vi "LQR.vi"() -> ()   [LabVIEW 2019]
uses:
  <vilib>/Platform/TimedLoop/XDataNode/timing_clust.ctl
  <vilib>/Platform/TimedLoop/XDataNode/nitl_modes.ctl
  <vilib>/Platform/TimedLoop/XDataNode/wakeup.ctl
  <vilib>/Simulation/Shared/_Datatypes/SIM SISO Transfer Function.ctl
  <vilib>/myRIO/Instrument Drivers/Onboard IO/AI/typedefs/AI Reference.ctl
  <vilib>/myRIO/Common/Instrument Driver Framework/Utilities/typedefs/myRIO Generic Hardware Reference.ctl
  <vilib>/myRIO/Common/Instrument Driver Framework/Utilities/typedefs/Hardware Version Enum.ctl
  <vilib>/myRIO/Common/Instrument Driver Framework/Utilities/typedefs/myRIO v1.0 Reference.ctl
  <vilib>/myRIO/Common/Instrument Driver Framework/Utilities/typedefs/Generic FPGA Reference.ctl
  <vilib>/myRIO/Common/Instrument Driver Framework/myRIO v1.0/AI/typedefs/AI Channels List.ctl
  <vilib>/myRIO/Common/Instrument Driver Framework/myRIO v1.0/AI/typedefs/AI Channels Enum.ctl
  <vilib>/myRIO/Common/Instrument Driver Framework/Utilities/typedefs/Analog Scaling Constants List.ctl
  <vilib>/myRIO/Common/Instrument Driver Framework/Utilities/typedefs/Analog Scaling Constants.ctl
  <vilib>/userDefined/High Color/nirio_resource_hc.ctl
  <vilib>/myRIO/Instrument Drivers/Onboard IO/AO/typedefs/AO Reference.ctl
  <vilib>/myRIO/Common/Instrument Driver Framework/myRIO v1.0/AO/typedefs/AO Channels List.ctl
  <vilib>/myRIO/Common/Instrument Driver Framework/myRIO v1.0/AO/typedefs/AO Channels Enum.ctl
  <vilib>/myRIO/Common/Instrument Driver Framework/Utilities/vis/Is FPGA Ref Available.vi
  <vilib>/myRIO/Common/Instrument Driver Framework/myRIO v1.0/AI/vis/myRIO v1.1 Open AI.vi
  <vilib>/myRIO/Instrument Drivers/Onboard IO/AI/vis/Read.vi
  <vilib>/Simulation/DiscreteLinear/Implementation/NILVSim Discrete Transfer Function Direct.llb/SIM Discrete Transfer Function Diagram (SISO).vi
  <vilib>/myRIO/Common/Instrument Driver Framework/myRIO v1.0/AO/vis/myRIO v1.1 Open AO.vi
  <vilib>/myRIO/Instrument Drivers/Onboard IO/AO/vis/Write.vi
  <vilib>/myRIO/Common/Instrument Driver Framework/Utilities/vis/Validate Channels.vi
  <vilib>/myRIO/Common/Instrument Driver Framework/myRIO v1.0/AI/vis/myRIO v1.0 Reserve AI.vi
  <vilib>/Simulation/ContinuousLinear/Implementation/Shared/SIM Transfer Function Support.llb/SIM TransferFunction Normalize to Buffer.vi
  <vilib>/Simulation/DiscreteLinear/Implementation/Shared/SIM Init Discrete States.vi
  <vilib>/Simulation/DiscreteLinear/Implementation/NILVSim Discrete Transfer Function Direct.llb/SIM Transfer Function Direct core (SISO).vi
  <vilib>/myRIO/Common/Instrument Driver Framework/myRIO v1.0/AO/vis/myRIO v1.0 Reserve AO.vi
  <vilib>/myRIO/Common/Instrument Driver Framework/myRIO v1.0/AI/vis/myRIO v1.0 Build MUX Configuration AI.vi
  <vilib>/myRIO/Common/Instrument Driver Framework/myRIO v1.0/Resource Manager/vis/myRIO v1.0 Reserve Channel List.vi
  <vilib>/Simulation/ContinuousLinear/Implementation/Shared/SIM Transfer Function Support.llb/SIM TransferFunction Normalize.vi
  <vilib>/myRIO/Common/Instrument Driver Framework/myRIO v1.0/AO/vis/myRIO v1.0 Build MUX Configuration AO.vi
  <vilib>/myRIO/Common/Instrument Driver Framework/myRIO v1.0/Resource Manager/vis/myRIO v1.0 Reserve Channel.vi
  <vilib>/myRIO/Common/Instrument Driver Framework/myRIO v1.0/Resource Manager/vis/myRIO v1.0 Unreserve Channel.vi
  <vilib>/Simulation/Implementation/Shared/SIM Polynomials.llb/SIM Remove Zero Coefficients (DBL).vi
  <vilib>/myRIO/Common/Instrument Driver Framework/myRIO v1.0/Resource Manager/vis/myRIO v1.0 Build Mutex Name.vi
  <vilib>/Simulation/Implementation/Shared/SIM Polynomials.llb/SIM Divide Polynomials (DBL).vi
  <vilib>/Simulation/Implementation/Shared/SIM BuildSimErr.vi
  <vilib>/Utility/VariantDataType/GetNumericInfo.vi
  <vilib>/Utility/error.llb/Error Cluster From Error Code.vi
  <vilib>/myRIO/Common/Instrument Driver Framework/myRIO v1.0/myRIO v1.1 Open.vi
  <vilib>/myRIO/Common/Instrument Driver Framework/myRIO v1.0/AI/vis/myRIO v1.0 Get Scaling Constants AI.vi
  <vilib>/myRIO/Common/Instrument Driver Framework/Utilities/vis/IO Manager.vi
  <vilib>/myRIO/Common/Instrument Driver Framework/Utilities/vis/Configuration Manager.vi
  <vilib>/myRIO/Common/Instrument Driver Framework/myRIO v1.0/myRIO v1.0 Close.vi
  <vilib>/myRIO/Common/Instrument Driver Framework/myRIO v1.0/AI/vis/myRIO v1.0 Read AI.vi
  <vilib>/myRIO/Common/Instrument Driver Framework/myRIO v1.0/AO/vis/myRIO v1.0 Get Scaling Constants AO.vi
  <vilib>/myRIO/Common/Instrument Driver Framework/myRIO v1.0/AO/vis/myRIO v1.0 Write AO.vi
  <vilib>/platform/TimedLoop/XDataNode/XDataNode.xnode
  <vilib>/Simulation/Implementation/XNodeFramework/SimXNode/SimX.xnode
  <vilib>/myRIO/Express VI/Onboard IO/AI/AI Express VI.xnode
  <vilib>/myRIO/Instrument Drivers/Onboard IO/AI/vis/myRIO AI Open.xnode
  <vilib>/myRIO/Express VI/Onboard IO/AO/AO Express VI.xnode
  <vilib>/myRIO/Instrument Drivers/Onboard IO/AO/vis/myRIO AO Open.xnode
  <vilib>/Platform/TimedLoop/XDataNode/XDNodeRunTimeDep.lvlib
  <vilib>/myRIO/Instrument Drivers/Onboard IO/AI/AI.lvlib
  <vilib>/myRIO/Instrument Drivers/Onboard IO/AO/AO.lvlib
  <vilib>/ptbypt/NI_PtbyPt.lvlib
panel:
  in  "amplitude":dbl=1.0 format="%0.2f"
  out "Impulse Pattern":dbl(graph)
  in  "D":dbl=7.3
  in  "P":dbl=5291.0
  in  "stopNoise":bool=TRUE
  in  "gain_noise":dbl=0.2
  out "uniform white noise":dbl(graph)=-0.031193239239623867
  in  "AmpWhitehNoise":dbl=1.0 format="%0.2f"
  out "Iteration Duration":i64(graph)=347
  in  "Max FRF current 0-1000mA":dbl=4.0
  in  "Stop FRF":bool=TRUE
  in  "esc":bool
  out "scope":cluster{dbl, dbl, dbl, dbl, dbl}(graph)={-8.303163599999976, 0.03990822535355048, -0.0, -8.32082689025263, 946.4168275057085}
  out "Current Output EM":dbl(graph)=0.03990822535355048
  in  "Stop EM + FRF":bool=TRUE
  out "left[V]":dbl=-0.0
  out "right[V]":dbl=-0.0
  out "um":dbl=376.9531636
  # "mA"
types:
  T1 = typedef "XDNodeRunTimeDep.lvlib/timing_clust.ctl" = cluster{"Expected End [f-1]":u64, "Actual End [f-1]":u64, "Finished Late? [f-1]":bool, "Expected End [i-1]":u64, "Actual End [i-1]":u64, "Finished Late? [i-1]":bool, "Expected Start [i]":u64, "Actual Start [i]":u64, "Expected Start [f]":u64, "Actual Start [f]":u64, "Source Name":string, "Structure Name":string, "Period":i64, "Deadline":i64, "Offset":i64, "Start":i64, "Priority":i32, "Timeout":i32, "Mode":T2, "Wakeup Reason":T3, "Error":errorcluster, "Source Type":string, "Secondary Source Type":string, "Global End Time":u64, "Global Start Time":u64, "Frame Duration":u64, "Iteration Duration":u64, "Assigned CPU":i32, "I/O Scan Engine Mode":u32}
  T2 = typedef "XDNodeRunTimeDep.lvlib/nitl_modes.ctl" = enum32{"No Change", "Process missed periods, maintain original phase", "Discard missed periods, maintain original phase", "Process missed periods, ignore original phase", "Discard missed periods, ignore original phase"}
  T3 = typedef "XDNodeRunTimeDep.lvlib/wakeup.ctl" = enum32{"Normal", "Aborted", "Asynchronous wakeup", "Timing source error", "Timed loop error", "Timeout"}
  T4 = typedef "SIM SISO Transfer Function.ctl" = cluster{"Numerator":dbl[], "Denominator":dbl[]}
  T5 = typedef "AI.lvlib/AI Reference.ctl" = cluster{"myRIO Reference":T6, "AI Channels List":T10, "AI Scaling Constants List":T12}
  T6 = typedef "myRIO Generic Hardware Reference.ctl" = cluster{"myRIO Model":T7, "myRIO Hardware Reference":T8}
  T7 = typedef "Hardware Version Enum.ctl" = enum16{"Unknown", "myRIO-1900", "myRIO-1950", "roboRIO", "NI ELVIS RIO CM", "ELVIS III"}
  T8 = typedef "myRIO v1.0 Reference.ctl" = cluster{"Generic FPGA Reference":T9, "Allow multiple opens":bool}
  T9 = typedef "Generic FPGA Reference.ctl" = refnum<k20>
  T10 = typedef "AI Channels List.ctl" = T11[]
  T11 = typedef "AI Channels Enum.ctl" = enum16{"Not Connected", "AudioIn/Left", "AudioIn/Right", "C/AI0", "C/AI1", "A/AI0", "A/AI1", "A/AI2", "A/AI3", "A/AI4", "A/AI5", "A/AI6", "A/AI7", "B/AI0", "B/AI1", "B/AI2", "B/AI3", "B/AI4", "B/AI5", "B/AI6", "B/AI7", "AI/AI0", "AI/AI1", "AI/AI2", "AI/AI3", "A/AI0 (DIFF)", "A/AI1 (DIFF)", "A/AI2 (DIFF)", "A/AI3 (DIFF)", "B/AI0 (DIFF)", "B/AI1 (DIFF)", "B/AI2 (DIFF)", "B/AI3 (DIFF)"}
  T12 = typedef "Analog Scaling Constants List.ctl" = T13[]
  T13 = typedef "Analog Scaling Constants.ctl" = cluster{"LSB Weight (Volts)":dbl, "Offset (Volts)":dbl, "Signed?":bool}
  T14 = typedef "nirio_resource_hc.ctl" = tag
  T15 = typedef "AO.lvlib/AO Reference.ctl" = cluster{"myRIO Reference":T6, "AO Channel List":T16, "AO Scaling Constant List":T12}
  T16 = typedef "AO Channels List.ctl" = T17[]
  T17 = typedef "AO Channels Enum.ctl" = enum16{"Not Connected", "AudioOut/Left", "AudioOut/Right", "C/AO0", "C/AO1", "A/AO0", "A/AO1", "B/AO0", "B/AO1"}
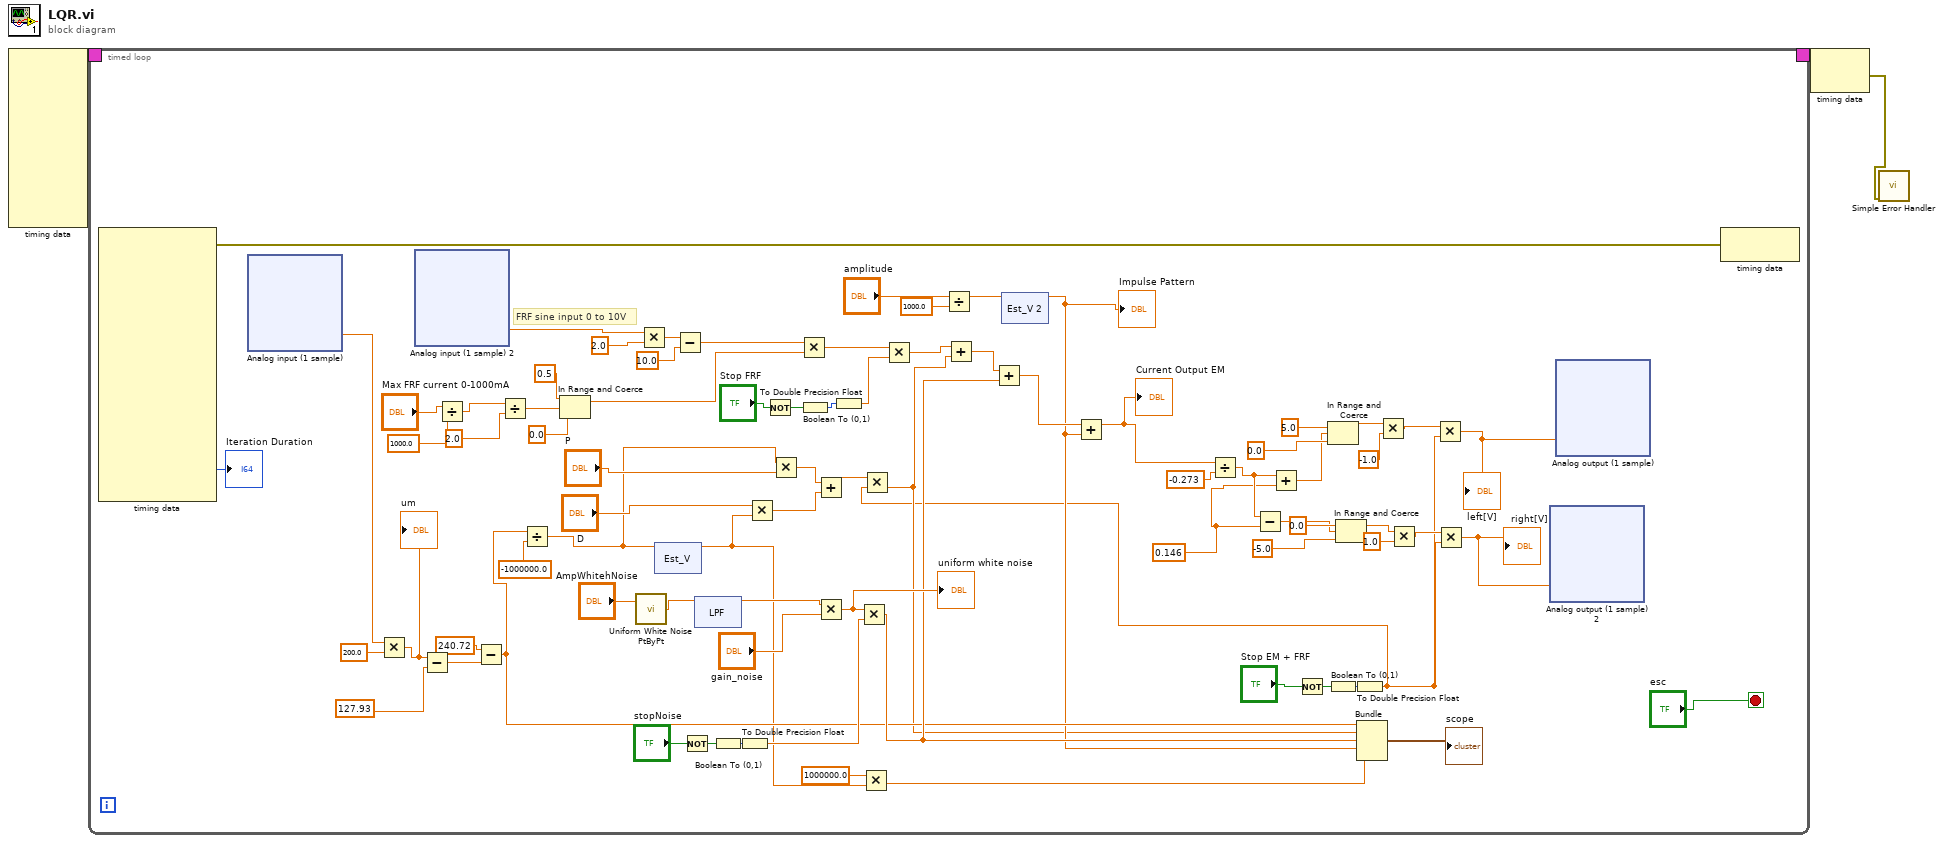
[diagram p0: block diagram]
diagram:
  n1 = node-c288() -> (w3:T1)  [unwired: 10 in]
  n2 = timed-loop {
    timing: w3 -> [_]
    timing-out: [_] -> w2
    stop <- "esc" stop-if-true
    w41 = 0.146 ("y")
    # "FRF sine input 0 to 10V"
    n3 = node-c288() -> (w82:errorcluster, →"Iteration Duration":i64)  [unwired: 1 in, 15 out]
    n4 = xnode "Analog input (1 sample)"() -> ("C/AI1 (AI1)"=w38:dbl)  [unwired: 1 in, 1 out]
    n5 = Multiply(x=w38, y=200.0) -> (x*y=w80:dbl)
    "um" <- w80
    n6 = xnode "Analog input (1 sample) 2"() -> ("C/AI0 (AI0)"=w59:dbl)  [unwired: 1 in, 1 out]
    n7 = Subtract(x=w80, y=127.93) -> (x-y=w79:dbl)
    n8 = Divide(x="Max FRF current 0-1000mA", y=1000.0) -> (x/y=w48:dbl)
    n9 = Subtract(x=240.72, y=w79) -> (x-y=w21:dbl)
    n10 = Divide(x=w48, y=2.0) -> (x/y=w52:dbl)
    n11 = Divide(x=w21, y=-1000000.0) -> (x/y=w11:dbl)
    n12 = In Range and Coerce(upper limit=0.5, x=w52, lower limit=0.0) -> (coerced(x)=w49:dbl)  [unwired: 1 out]
    n13 = call <vilib>:"Uniform White Noise PtByPt.vi"("amplitude"="AmpWhitehNoise") -> ("uniform white noise"=w31:dbl)  [unwired: 2 in]
    n14 = Multiply(x=w59, y=2.0) -> (x*y=w57:dbl)
    n15 = xnode "Est_V"("input u(k)"=w11) -> ("output y(k)"=w12:dbl)  [unwired: 2 in, 1 out]
    n16 = Subtract(x=w57, y=10.0) -> (x-y=w54:dbl)
    n17 = Not(x="stopNoise") -> (.not. x?=w29:bool)
    n18 = xnode "LPF"("input u(k)"=w31) -> ("output y(k)"=w28:dbl)  [unwired: 2 in, 1 out]
    n19 = Boolean To (0,1)(Boolean=w29) -> (0, 1=w30:i16)
    n20 = To Double Precision Float(number=w30) -> (double precision float=w25:dbl)
    n21 = Multiply(x="D", y=w12) -> (x*y=w19:dbl)
    n22 = Not(x="Stop FRF") -> (.not. x?=w62:bool)
    n23 = Multiply(x=w11, y="P") -> (x*y=w20:dbl)
    n24 = Multiply(x=w54, y=w49) -> (x*y=w55:dbl)
    n25 = Boolean To (0,1)(Boolean=w62) -> (0, 1=w61:i16)
    n26 = Add(x=w20, y=w19) -> (x+y=w5:dbl)
    n27 = Multiply(x=w28, y="gain_noise") -> (x*y=w24:dbl)
    "uniform white noise" <- w24
    n28 = To Double Precision Float(number=w61) -> (double precision float=w60:dbl)
    n29 = Multiply(x=w24, y=w25) -> (x*y=w23:dbl)
    n30 = Multiply(x=1000000.0, y=w12) -> (x*y=w8:dbl)
    n31 = Multiply(x=w55, y=w60) -> (x*y=w64:dbl)
    n32 = Divide(x="amplitude", y=1000.0) -> (x/y=w14:dbl)
    n33 = xnode "Est_V 2"("input u(k)"=w14) -> ("output y(k)"=w9:dbl)  [unwired: 2 in, 1 out]
    "Impulse Pattern" <- w9
    n34 = Not(x="Stop EM + FRF") -> (.not. x?=w67:bool)
    n35 = Boolean To (0,1)(Boolean=w67) -> (0, 1=w69:i16)
    n36 = To Double Precision Float(number=w69) -> (double precision float=w4:dbl)
    n37 = Multiply(x=w5, y=w4) -> (x*y=w6:dbl)
    n38 = Add(x=w64, y=w6) -> (x+y=w22:dbl)
    n39 = Add(x=w22, y=w23) -> (x+y=w16:dbl)
    n40 = Add(x=w16, y=w9) -> (x+y=w10:dbl)
    "Current Output EM" <- w10
    n41 = Divide(x=w10, y=-0.273) -> (x/y=w42:dbl)
    n42 = Subtract(x=w42, y=w41) -> (x-y=w43:dbl)
    n43 = Add(x=w42, y=w41) -> (x+y=w44:dbl)
    n44 = In Range and Coerce(upper limit=5.0 ("x"), x=w44, lower limit=0.0) -> (coerced(x)=w35:dbl)  [unwired: 1 out]
    n45 = In Range and Coerce(upper limit=0.0 ("x"), x=w43, lower limit=-5.0) -> (coerced(x)=w72:dbl)  [unwired: 1 out]
    n46 = Bundle(w21, w6, w23, "output y(k)"=w9, w8) -> (→"scope":cluster{dbl, dbl, dbl, "output y(k)":dbl, dbl})  [unwired: 1 in]
    n47 = Multiply(x=w35, y=-1.0) -> (x*y=w40:dbl)
    n48 = Multiply(x=w72, y=1.0) -> (x*y=w39:dbl)
    n49 = Multiply(x=w40, y=w4) -> (x*y=w37:dbl)
    "left[V]" <- w37
    n50 = Multiply(x=w39, y=w4) -> (x*y=w36:dbl)
    "right[V]" <- w36
    n51 = xnode "Analog output (1 sample) 2"("C/AO1 (AO1)"=w36) -> ()  [unwired: 1 in, 1 out]
    n52 = xnode "Analog output (1 sample)"("C/AO0 (AO0)"=w37) -> ()  [unwired: 1 in, 1 out]
    n53 = node-c288(w82) -> ()  [unwired: 1 out]
  }
  n54 = node-c288(w2) -> (w1:errorcluster)
  n55 = call <vilib>:"Simple Error Handler.vi"("error in (no error)"=w1) -> ()  [unwired: 4 in, 5 out]
